vi "Test Get Named Range Values (Boolean).vi"(11 "Test Case In":refnum<class "Test Open Xml.lvclass">) -> (0 "error out":errorcluster, 3 "Test Case Out":refnum<class "Test Open Xml.lvclass">)   [LabVIEW 2020, in "Test Open Xml.lvclass"]
uses:
  Test Open Xml.lvclass
  C:/Program Files/National Instruments/LabVIEW 2025/vi.lib/Astemes/LUnit/Test Case.lvclass
  <vilib>/Astemes/LUnit/Test Case.lvclass/Test Case.ctl
  Test Open Xml.lvclass/Test Open Xml.ctl
  e7d09ce7-04db-40ce-9c4e-a78b31ec9fe8.vi
  Source/Open Xml.lvlib
  50f757ab-2d74-46a0-bdd7-e6f0543e2c81.vi
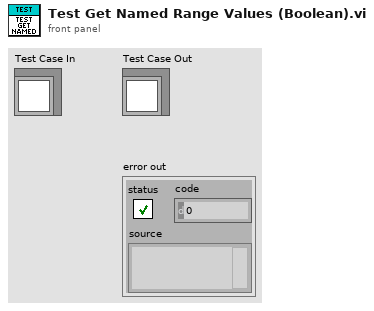
[diagram p1: front panel]
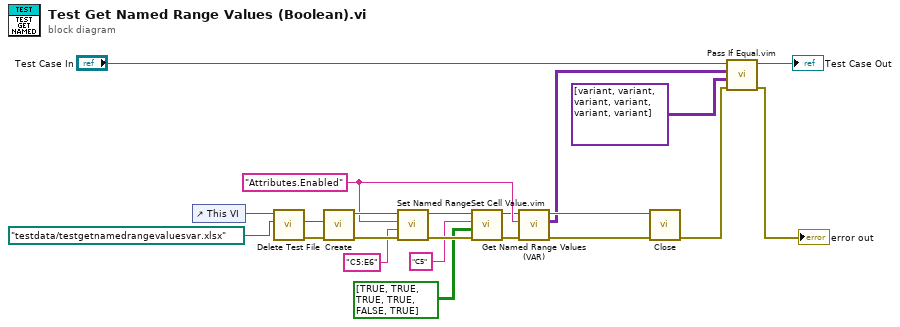
[diagram p0: block diagram]
diagram:
  w8 = "Attributes.Enabled" ("Sheet Name")
  n1 = control-ref of="This VI"() -> (w13:refnum<vi>)
  n2 = call "Delete Test File.vi"("name or relative path"=path "testdata/testgetnamedrangevaluesvar.xlsx", "VI in"=w13) -> ("error out"=w11:errorcluster, "deleted path"=w12:path)  [unwired: 8 in]
  n3 = call "Create.vi"("error in"=w11, "Path"=w12) -> ("error out"=w19:errorcluster, "SpreadsheetDoc"=w9:refnum<k24>)  [unwired: 8 in]
  n4 = call "Set Named Range.vi"("error in"=w19, "Cell Range"="C5:E6" ("Cell Address"), "Named Range Identifier"=w8, "SpreadsheetDoc in"=w9) -> ("error out"=w10:errorcluster, "SpreadsheetDoc out"=w6:refnum<k24>)  [unwired: 6 in]
  n5 = call "Set Cell Value.vim"("error in"=w10, "Value"=bool[][] [[TRUE, TRUE, TRUE], [TRUE, FALSE, TRUE]], "Cell Address"="C5", "SpreadsheetDoc in"=w6) -> ("error out"=w7:errorcluster, "SpreadsheetDoc out"=w5:refnum<k24>)  [unwired: 6 in]
  n6 = call "Get Named Range Values (VAR).vi"("error in"=w7, "Named Range Identifier"=w8, "SpreadsheetDoc in"=w5) -> ("error out"=w18:errorcluster, "Cells"=w15:variant[][], "SpreadsheetDoc out"=w16:refnum<k24>)  [unwired: 6 in]
  n7 = call "Close.vi"("error in"=w18, "SpreadsheetDoc"=w16) -> ("error out"=w17:errorcluster)  [unwired: 9 in]
  n8 = call "Pass If Equal.vim"("error in (no error)"=w17, "Actual"=variant[][] [[variant(bool TRUE), variant(bool TRUE), variant(bool TRUE)], [variant(bool TRUE), variant(bool FALSE), variant(bool TRUE)]] ("Cells"), "Expected"=w15, "LUnit Test Case In"="Test Case In") -> ("error out"=→"error out":errorcluster, "LUnit Test Case Out"=→"Test Case Out":refnum<class "Test Open Xml.lvclass">)  [unwired: 6 in]
